vi "testAssertionFailureMessage.vi"() -> ()   [LabVIEW 2019, in "AssertionTest.lvlib" / "AssertNotEquals.lvlib"]
uses:
  AssertNotEquals.lvlib
  e79a45c8-443a-418e-8093-4721675f49db.vi
  Constraint/IsEqual/IsEqual.lvclass
  C:/Users/de200256/Code/LVUnit/Constraint/Constraint/Constraint.lvclass
  Constraint/IsEqual/Create.vi
  Constraint/LogicalNot/LogicalNot.lvclass
  Constraint/UnaryOperator/UnaryOperator.lvclass
  Assertion/Assertion.lvlib
panel:
  out "error out":errorcluster
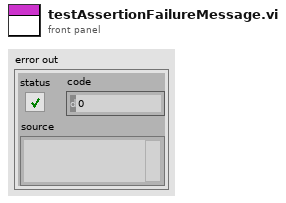
[diagram p1: front panel]
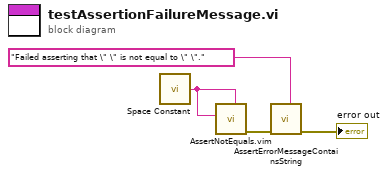
[diagram p0: block diagram]
diagram:
  n1 = call <vilib>:"Space Constant.vi"() -> ("String"=w1:string)
  n2 = call "AssertNotEquals.vim"("Expected"=w1, "Actual"=w1) -> ("error out"=w4:errorcluster)  [unwired: 9 in]
  n3 = call "AssertErrorMessageContainsString.vi"("Expected"="Failed asserting that \" \" is not equal to \" \"." ("y"), "error in (no error)"=w4) -> ("error out"=→"error out":errorcluster)  [unwired: 9 in]
